vi "TORC-TapeMeasureGlobal.vi"() -> ()   [LabVIEW 2014]
doc: "One of the VIs created by TORC 2137 to control the tape measure.\n\nThis is a set of two global variables; the first is the value read by the tape measure encoder, which is used by the code in Autonomous to compare current and target positions and move the tape measure. The second is the value written to by the Autonomous and Teleop code, which is read in Timed Tasks and sets the motor value (between -1 and 1) , actually moving the motor.\n\nPlease do not modify or read these values in your code unless absolutely neccessary."
panel:
  in  "TORCTapeMeasureMotor":dbl
  in  "TORCTapeMeasureEncoder":dbl
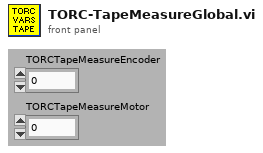
[diagram p1: front panel]
diagram:
